vi "PH_Beckhoff_StepMot.PC set Axis Settings.vi"(0 "VI in":refnum<vi>, 2 "Axis Settings":T1, 3 "Axis":i32, 5 "error in (no error)":errorcluster) -> (14 "VI out":refnum<vi>, 17 "Settings changed?":bool, 19 "error out":errorcluster)   [LabVIEW 2014, in "PH_Beckhoff_StepMot.lvlib"]
uses:
  PH_Beckhoff_StepMot.lvlib
  PH_Beckhoff_StepMot.Axis Cluster.ctl
  non_GPL/instr.lib/Beckhoff/Specials/Step Motor Klemmen/Beckhoff.Step Motor - Motor Configuration.ctl
  non_GPL/instr.lib/Beckhoff/Read and Write Register/Step Motor Klemmen/Beckhoff.Step Motor - Feature Register 1.ctl
  non_GPL/instr.lib/Beckhoff/Read and Write Register/Step Motor Klemmen/Beckhoff.Step Motor - Feature Register 2.ctl
  non_GPL/instr.lib/Beckhoff/Beckhoff - Driver np.lvlib
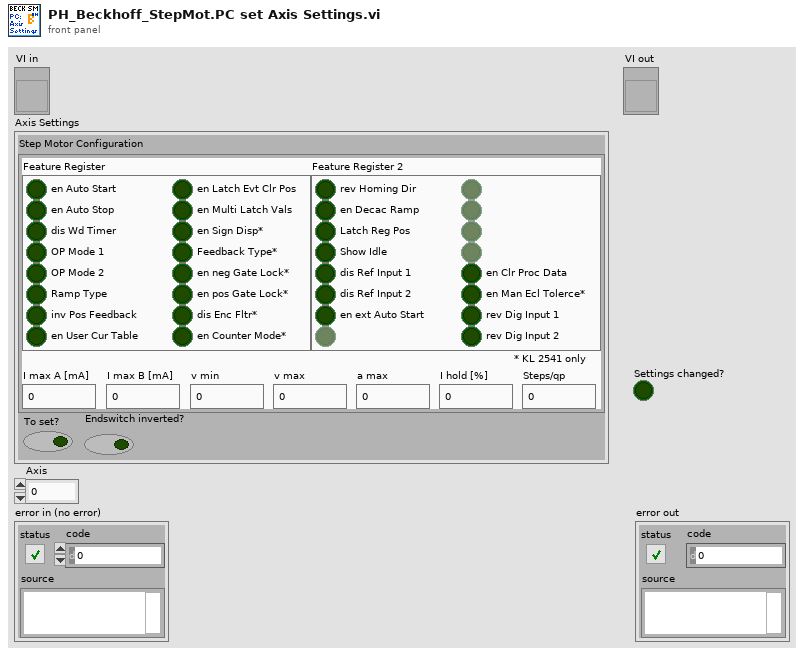
[diagram p1: front panel]
types:
  T1 = typedef "PH_Beckhoff_StepMot.lvlib/PH_Beckhoff_StepMot.Axis Cluster.ctl" = cluster{"Step Motor Configuration":T2, "To set?":bool, "Endswitch inverted?":bool}
  T2 = typedef "Beckhoff - Driver np.lvlib/Beckhoff.Step Motor - Motor Configuration.ctl" = cluster{"Feature Register":T3, "I max A [mA]":dbl, "I max B [mA]":dbl, "v min":u32, "v max":u32, "a max":u32, "I hold [%]":u32, "Steps/qp":u32, "Feature Register 2":T4}
  T3 = typedef "Beckhoff - Driver np.lvlib/Beckhoff.Step Motor - Feature Register 1.ctl" = cluster{"en Auto Start":bool, "en Auto Stop":bool, "dis Wd Timer":bool, "OP Mode 1":bool, "OP Mode 2":bool, "Ramp Type":bool, "inv Pos Feedback":bool, "en User Cur Table":bool, "en Latch Evt Clr Pos":bool, "en Multi Latch Vals":bool, "en Sign Disp*":bool, "Feedback Type*":bool, "en neg Gate Lock*":bool, "en pos Gate Lock*":bool, "dis Enc Fltr*":bool, "en Counter Mode*":bool}
  T4 = typedef "Beckhoff - Driver np.lvlib/Beckhoff.Step Motor - Feature Register 2.ctl" = cluster{"rev Homing Dir":bool, "en Decac Ramp":bool, "Latch Reg Pos":bool, "Show Idle":bool, "dis Ref Input 1":bool, "dis Ref Input 2":bool, "en ext Auto Start":bool, "N/A":bool, "N/A":bool, "N/A":bool, "N/A":bool, "N/A":bool, "en Clr Proc Data":bool, "en Man Ecl Tolerce*":bool, "rev Dig Input 1":bool, "rev Dig Input 2":bool}
  T5 = typedef "PH_Beckhoff_StepMot.lvlib/PH_Beckhoff_StepMot.i attribute.ctl" = cluster{"Axes Settings":T1[], "GUI Refs":cluster{"Axes Settings":refnum<vi>, "Stati":refnum<vi>}, "Get Beckhoff Settings":bool}
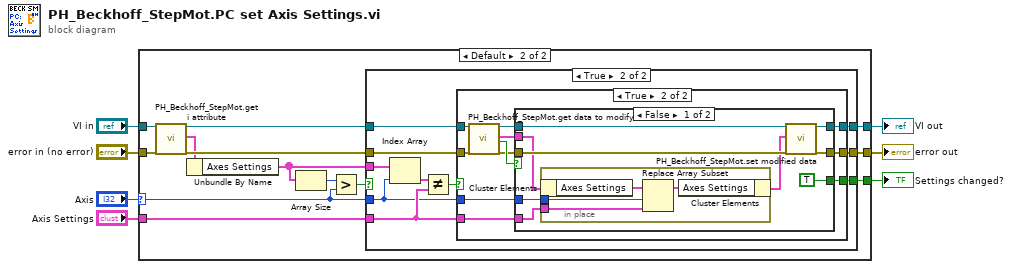
[diagram p0: block diagram]
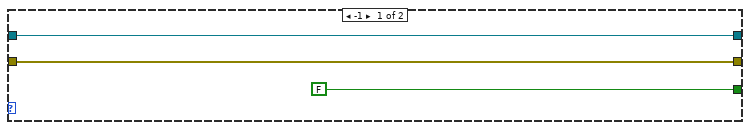
[diagram p2: hidden frame]
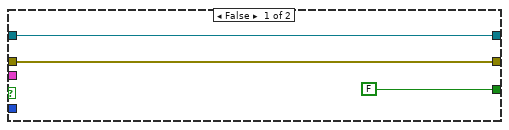
[diagram p3: hidden frame]
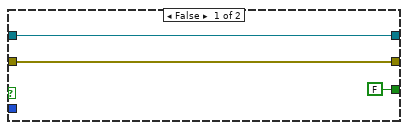
[diagram p4: hidden frame]
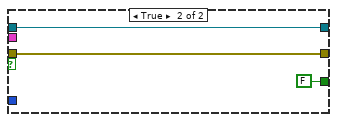
[diagram p5: hidden frame]
diagram:
  n1 = case shown="Default" "Axis" {
    selector: "Axis" -> [_ w12]
    tunnel: [w10 w23] -> w7
    tunnel: [w9 w22] -> w6
    tunnel: "error in (no error)" -> [w9 w21]
    tunnel: "VI in" -> [w10 w19]
    tunnel: "Axis Settings" -> [_ w16]
    tunnel: [FALSE w15] -> w2
    frame -1 {
    }
    frame Default {
      n2 = call "PH_Beckhoff_StepMot.get i attribute.vi"("i ref in"=w19, "error in (no error)"=w21) -> ("i ref out"=w18:refnum<vi>, "i attribute"=w17:T5, "error out"=w20:errorcluster)  [unwired: 15 in]
      n3 = Unbundle By Name(w17) -> ("Axes Settings"=w14:T1[])
      n4 = Array Size(array=w14) -> (size(s)=w13:i32)
      n5 = Greater?(x=w13, y=w12) -> (0:w11:bool)
      n6 = case shown="True" w11 {
        tunnel: [w26 w36] -> w23
        tunnel: [w25 w35] -> w22
        tunnel: w20 -> [w25 w34]
        tunnel: w18 -> [w26 w33]
        tunnel: w16 -> [_ w30]
        tunnel: [FALSE w29] -> w15
        tunnel: w14 -> [_ w28]
        tunnel: w12 -> [_ w27]
        frame False {
        }
        frame True {
          n7 = Index Array(array=w28, index=w27) -> (element=w32:T1)
          n8 = Not Equal?(x=w32, y=w30) -> (x != y?=w31:bool)
          n9 = case shown="True" w31 {
            tunnel: [w39 w48] -> w36
            tunnel: [w38 w46] -> w35
            tunnel: w34 -> [w38 w44]
            tunnel: w33 -> [w39 w43]
            tunnel: w30 -> [_ w42]
            tunnel: w27 -> [_ w41]
            tunnel: [FALSE w40] -> w29
            frame False {
            }
            frame True {
              n10 = call "PH_Beckhoff_StepMot.get data to modify.vi"("i ref in"=w43, "error in (no error)"=w44) -> ("i ref out"=w47:refnum<vi>, "i attribute"=w50:T5, "timed out"=w49:bool, "error out"=w45:errorcluster)  [unwired: 14 in]
              n11 = case shown="False" w49 {
                tunnel: w45 -> [w59 w65]
                tunnel: [w58 w65] -> w46
                tunnel: w47 -> [w57 w66]
                tunnel: [w56 w66] -> w48
                tunnel: w50 -> [w54 _]
                tunnel: w42 -> [w52 _]
                tunnel: w41 -> [w53 _]
                tunnel: [TRUE FALSE] -> w40
                frame False {
                  n12 = in-place {
                    in-place-border: w53 -> [w62]
                    in-place-border: w52 -> [w61]
                    n13 = in-place-cluster #1(w54) -> ("Axes Settings"=w63:T1[])
                    n14 = Replace Array Subset(array=w63, new element=w61, index=w62) -> (w60:T1[])
                    n15 = in-place-cluster #1("Axes Settings"=w60) -> (w51:T5)
                  }
                  n16 = call "PH_Beckhoff_StepMot.set modified data.vi"("i ref in"=w57, "i attribute"=w51, "error in (no error)"=w59) -> ("i ref out"=w56:refnum<vi>, "error out"=w58:errorcluster)  [unwired: 15 in]
                }
                frame True {
                }
              }
            }
          }
        }
      }
    }
  }
  "VI out" <- w7
  "error out" <- w6
  "Settings changed?" <- w2
